vi "Read Values.vi"(7 "read subset":T2, 8 "error in":errorcluster, 9 "channel names":string[](array[string]), 10 "group names":string[](array[string]), 11 "tdms file":refnum<k34>) -> (0 "error out":errorcluster, 1 "waveform timestamps = 0":bool, 2 "waveform values":waveform(dbl)[](array[waveform]), 3 "tdms file out":refnum<k34>, 4 "table values":T1, 6 "widest value strings":string[](array[string]))   [LabVIEW 2020, in "TdmsFileViewer.lvlib"]
uses:
  TdmsFileViewer.lvlib
  Table Components.ctl
  38c91d4d-4d0d-4045-a82e-4a749029f5f0.vi
  <vilib>/ProgressBar/Progress Bar Dialog.lvclass
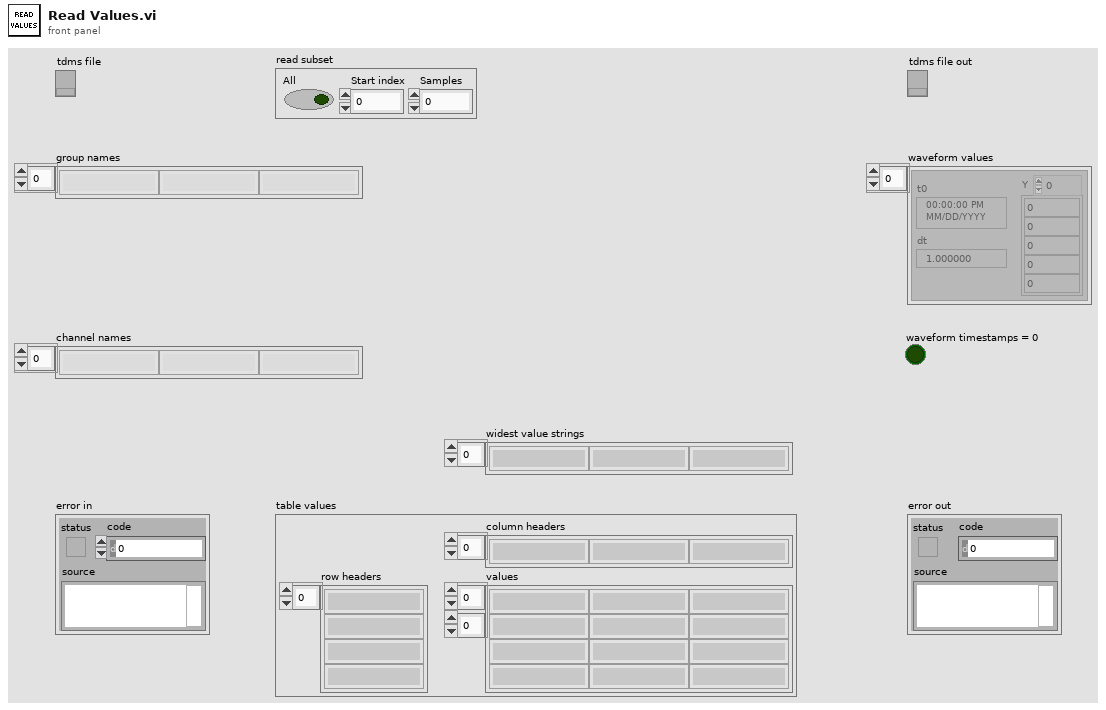
[diagram p1: front panel]
types:
  T1 = typedef "TdmsFileViewer.lvlib/Table Components.ctl" = cluster{"column headers":string[], "row headers":string[], "values":string[][]}
  T2 = cluster{"All":bool, "Start index":i64, "Samples":i64}
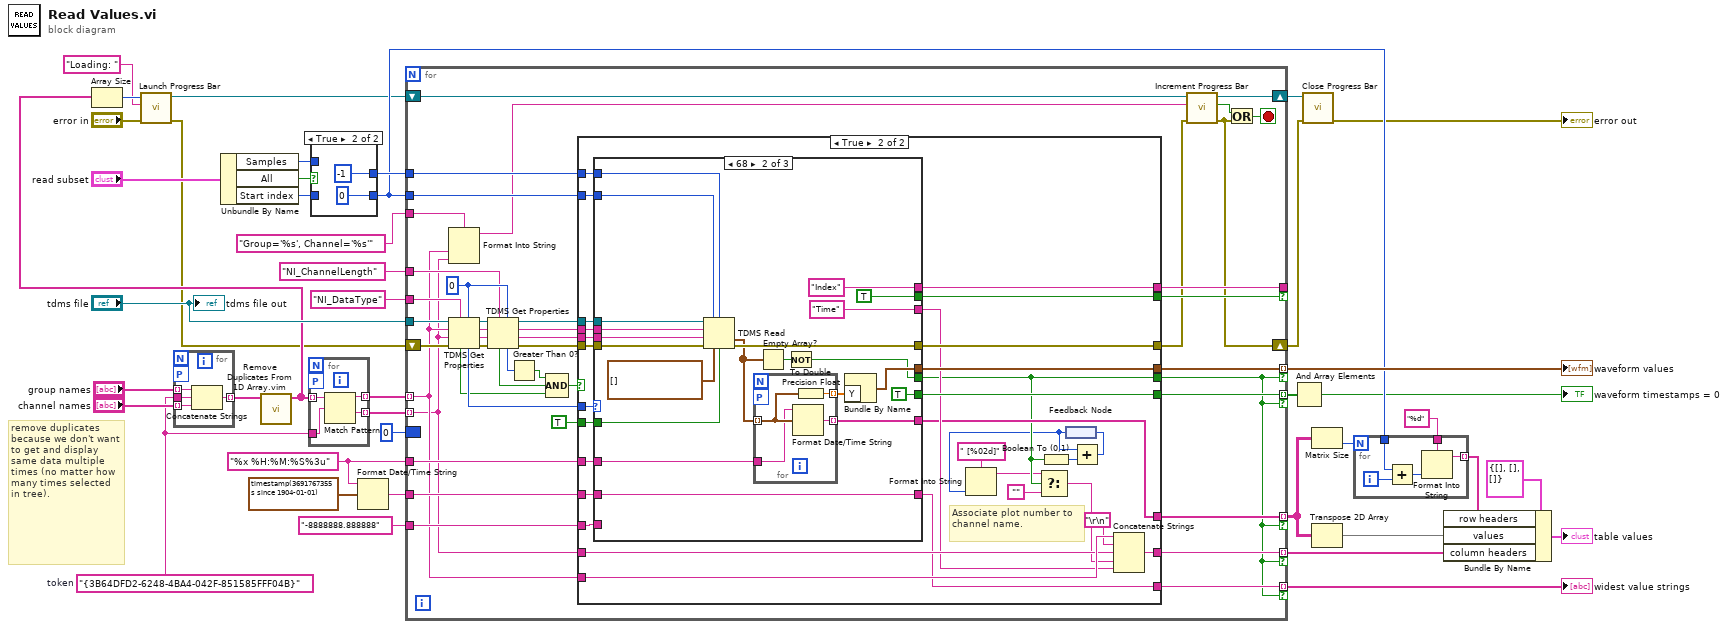
[diagram p0: block diagram]
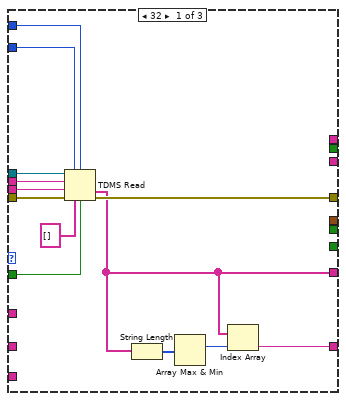
[diagram p4: hidden frame]
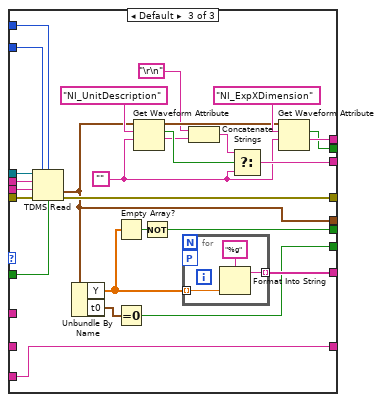
[diagram p5: hidden frame]
diagram:
  w12 = "{3B64DFD2-6248-4BA4-042F-851585FFF04B}"  # token
  w25 = "%x %H:%M:%S%3u" ("time format string (%c)")
  # "remove duplicates because we don't want to get and display same data multiple times (no matter how many times selected in tree)."
  n1 = for {
    workers-P: _ -> [_]
    tunnel: "group names" -> [w46] mode=indexing
    tunnel: "channel names" -> [w45] mode=indexing
    tunnel: w12 -> [w44]
    tunnel: [w43] -> w15 mode=indexing
    n2 = Concatenate Strings(w46, w44, w45) -> (w43:string)
  }
  n3 = Unbundle By Name("read subset") -> ("Samples"=w35:i64, "All"=w34:bool, "Start index"=w40:i64)
  n4 = call "Remove Duplicates From 1D Array.vim"("array"=w15) -> ("array with duplicates removed"=w4:string[])  [unwired: 10 in]
  n5 = Array Size(array=w4) -> (size(s)=w10:i32)
  n6 = call <vilib>:"Launch Progress Bar.vi"("error in (no error)"="error in", "Main Title (\"Working...\")"="Loading: " ("Main Title (\"Working...\")"), "Total Count"=w10) -> ("error out"=w2:errorcluster, "Progress Bar Dialog"=w8:refnum<class "Progress Bar Dialog.lvclass">)  [unwired: 7 in]
  n7 = for {
    tunnel: w4 -> [w50] mode=indexing
    workers-P: _ -> [_]
    tunnel: [w49] -> w14 mode=indexing
    tunnel: [w48] -> w13 mode=indexing
    tunnel: w12 -> [w47]
    n8 = Match Pattern(string=w50, regular expression=w47) -> (before substring=w49:string, after substring=w48:string)  [unwired: 1 in, 2 out]
  }
  n9 = case shown="True" w34 {
    tunnel: [w52 i64 -1 ("count (-1: all)")] -> w41
    tunnel: w40 -> [w51 _]
    tunnel: w35 -> [w52 _]
    tunnel: [w51 u64 0 ("t")] -> w32
    frame False {
    }
    frame True {
    }
  }
  n10 = Format Date/Time String(time format string (%c)=w25, seconds (now)=timestamp(3691767355.888 s since 1904-01-01)) -> (date/time string=w23:string)  [unwired: 1 in]
  n11 = for {
    tunnel: w32 -> [w94]
    tunnel: w41 -> [w93]
    tunnel: [w92] -> w39 mode=indexing if=w67
    tunnel: w13 -> [w61] mode=indexing
    shift-right: [w55] -> w1
    shift-left: w2 -> [w97]
    tunnel: w14 -> [w62] mode=indexing
    tunnel: [w91] -> _ if=w75
    tunnel: "NI_DataType" ("property name") -> [w77]
    tunnel: "NI_ChannelLength" ("property name") -> [w76]
    tunnel: [w74] -> w27 mode=indexing if=w67
    tunnel: w25 -> [w73]
    tunnel: w23 -> [w72]
    tunnel: [w71] -> w21 mode=indexing if=w67
    tunnel: "-8888888.888888" ("date/time string") -> [w70]
    tunnel: [w69] -> w20 mode=indexing if=w67
    tunnel: [w68] -> w19 mode=indexing if=w67
    tunnel: "tdms file" -> [w66]
    border: u16 0 -> [_]
    shift-right: [w63] -> w7
    shift-left: w8 -> [w64]
    tunnel: "Group='%s', Channel='%s'" ("format string") -> [w60]
    stop <- w58 stop-if-true
    w78 = u16 0
    n12 = Format Into String(format string=w60, w62, w61) -> (resulting string=w59:string)  [unwired: 2 in, 1 out]
    n13 = TDMS Get Properties(5:w78, 7:w77, 8:w97, 9:w61, 10:w62, 11:w66) -> (0:w96:errorcluster, 1:w85:string, 2:w86:string, 3:w89:refnum<k34>, 4:w90:u16, 6:w81:bool)
    n14 = TDMS Get Properties(5:w78, 7:w76, 8:w96, 9:w85, 10:w86, 11:w89) -> (0:w95:errorcluster, 1:w88:string, 2:w87:string, 3:w65:refnum<k34>, 4:w84:u16, 6:w82:bool)
    n15 = Greater Than 0?(x=w84) -> (x > 0?=w83:bool)
    n16 = Compound Arithmetic op=AND(w83, w82, w81) -> (w80:bool)
    n17 = case shown="True" w80 {
      tunnel: w94 -> [_ w127]
      tunnel: w93 -> [_ w126]
      tunnel: [w98 w128] -> w56
      tunnel: [_ w120] -> w92
      tunnel: [_ w125] -> w91
      tunnel: w65 -> [_ w124]
      tunnel: w95 -> [w98 w129]
      tunnel: w87 -> [_ w123]
      tunnel: w88 -> [_ w122]
      tunnel: w90 -> [_ w121]
      tunnel: w62 -> [_ w119]
      tunnel: w61 -> [_ w118]
      tunnel: [_ w108] -> w69
      tunnel: TRUE ("return channels in file order? (F)") -> [_ w117]
      tunnel: [_ w116] -> w75
      tunnel: [_ w104] -> w67
      tunnel: [_ w115] -> w74
      tunnel: w73 -> [_ w114]
      tunnel: w72 -> [_ w111]
      tunnel: [_ w109] -> w71
      tunnel: w70 -> [_ w110]
      tunnel: [_ w107] -> w68
      frame False {
      }
      frame True {
        # "Associate plot number to channel name."
        n18 = case shown="68" w121 {
          tunnel: w127 -> [w135 w157 w192]
          tunnel: w126 -> [w134 w158 w191]
          tunnel: [w141 w162 w193] -> w128
          tunnel: [w132 w161 w186] -> w107
          tunnel: [_ w156 w169] -> w120
          tunnel: [_ "Index" w185] -> w125
          tunnel: w124 -> [w140 w143 w189]
          tunnel: w129 -> [w142 w163 w194]
          tunnel: w123 -> [w139 w155 w188]
          tunnel: w122 -> [w138 w160 w187]
          tunnel: w117 -> [w136 w154 w184]
          tunnel: [_ TRUE w183] -> w116
          tunnel: [_ w148 w180] -> w104
          tunnel: [_ TRUE w178] -> w115
          tunnel: w114 -> [_ w146 _]
          tunnel: [_ "Time" w172] -> w112
          tunnel: w111 -> [_ w144 _]
          tunnel: [w130 w144 w170] -> w109
          tunnel: w110 -> [_ _ w170]
          frame 32 {
            n19 = TDMS Read(0:w140, 1:w135, 2:w134, 5:w139, 7:w138, 11:w142, 12:string[] [], 13:w136) -> (10:w132:string[], 15:w141:errorcluster)  [unwired: 4 out]
            n20 = String Length(string=w132) -> (length=w133:i32[])
            n21 = Array Max & Min(array=w133) -> (max index (indices)=w131:i32)  [unwired: 3 out]
            n22 = Index Array(array=w132, index=w131) -> (element=w130:string)
          }
          frame 68 {
            n23 = TDMS Read(0:w143, 1:w157, 2:w158, 5:w155, 7:w160, 11:w163, 12:timestamp[] [], 13:w154) -> (10:w150:timestamp[], 15:w162:errorcluster)  [unwired: 4 out]
            n24 = for {
              tunnel: [w167] -> w161 mode=indexing
              tunnel: w150 -> [w166] mode=indexing
              tunnel: [w165] -> w153 mode=indexing
              tunnel: w146 -> [w164]
              workers-P: _ -> [_]
              n25 = Format Date/Time String(time format string (%c)=w164, seconds (now)=w166) -> (date/time string=w167:string)  [unwired: 1 in]
              n26 = To Double Precision Float(number=w166) -> (double precision float=w165:dbl)
            }
            n27 = Empty Array?(array=w150) -> (empty?=w149:bool)
            n28 = Not(x=w149) -> (.not. x?=w148:bool)
            n29 = Bundle By Name("Y"=w153) -> (w156:waveform(dbl))  [unwired: 1 in]
          }
          frame Default {
            w171 = ""
            n30 = TDMS Read(0:w189, 1:w192, 2:w191, 5:w188, 7:w187, 11:w194, 13:w184) -> (10:w169:waveform(dbl), 15:w193:errorcluster)  [unwired: 1 in, 4 out]
            n31 = Unbundle By Name(w169) -> ("Y"=w182:dbl[], "t0"=w179:timestamp)
            n32 = Empty Array?(array=w182) -> (empty?=w181:bool)
            n33 = Equal To 0?(x=w179) -> (x = 0?=w178:bool)
            n34 = Get Waveform Attribute(5:w171, 6:"NI_UnitDescription" ("name"), 7:w169) -> (1:w173:string, 2:w175:bool, 3:w177:waveform(dbl))  [unwired: 1 in, 1 out]
            n35 = Not(x=w181) -> (.not. x?=w180:bool)
            n36 = for {
              tunnel: w182 -> [w197] mode=indexing
              tunnel: [w196] -> w186 mode=indexing
              workers-P: _ -> [_]
              n37 = Format Into String(format string="%g", w197) -> (resulting string=w196:string)  [unwired: 2 in, 1 out]
            }
            n38 = Concatenate Strings("\r\n", w173) -> (w174:string)
            n39 = Select(t=w174, s=w175, f=w171) -> (s? t:f=w172:string)
            n40 = Get Waveform Attribute(5:w171, 6:"NI_ExpXDimension" ("name"), 7:w177) -> (1:w185:string, 2:w183:bool)  [unwired: 1 in, 2 out]
          }
        }
        n41 = Boolean To (0,1)(Boolean=w104) -> (0, 1=w103:i16)
        n42 = feedback #1() -> (w102:u16)
        n43 = Format Into String(format string=" [%02d]", w102) -> (resulting string=w100:string)  [unwired: 2 in, 1 out]
        n44 = Select(t=w100, s=w104, f="") -> (s? t:f=w99:string)
        n45 = Add(x=w102, y=w103) -> (x+y=w101:u16)
        n46 = feedback-in #1(w101) -> ()
        n47 = Concatenate Strings(w119, "\r\n", w118, w99, w112) -> (w108:string)
      }
    }
    n48 = call <vilib>:"Increment Progress Bar.vi"("error in (no error)"=w56, "Step Name (\"\")"=w59, "Progress Bar Dialog in"=w64) -> ("error out"=w55:errorcluster, "Cancelled?"=w57:bool, "Progress Bar Dialog out"=w63:refnum<class "Progress Bar Dialog.lvclass">)  [unwired: 6 in]
    n49 = Or(x=w57, y=w55) -> (x .or. y?=w58:bool)
  }
  "waveform values" <- w39
  "widest value strings" <- w21
  n50 = And Array Elements(Boolean array=w27) -> (logical AND=→"waveform timestamps = 0":bool)
  n51 = call <vilib>:"Close Progress Bar.vi"("error in (no error)"=w1, "Progress Bar Dialog"=w7) -> ("error out"=→"error out":errorcluster)  [unwired: 9 in]
  n52 = Matrix Size(0:w19) -> (2:w36:i32)  [unwired: 1 out]
  n53 = Transpose 2D Array(2D array=w19) -> (transposed array=w30:string[][])
  n54 = for {
    N: w36 -> [_]
    tunnel: [w202] -> w31 mode=indexing
    tunnel: "%d" ("format string") -> [w199]
    tunnel: w32 -> [w198]
    i -> [w201]
    n55 = Add(x=w198, y=w201) -> (x+y=w200:u64)
    n56 = Format Into String(format string=w199, w200) -> (resulting string=w202:string)  [unwired: 2 in, 1 out]
  }
  n57 = Bundle By Name(cluster=T1 {"column headers"=[], "row headers"=[], "values"=[]}, "row headers"=w31, "values"=w30, "column headers"=w20) -> (→"table values":T1)
  "tdms file out" <- "tdms file"
